vi "Read (Math).vi"(0 "VISA resource name":refnum<visa-resource-name>, 1 "Sample Count (1)":i32=1, 5 "Math Operation (0: Power)":u16(ring) items=["Power", "Offset Compensated Ohms", "Resistor Voltage Coefficient", "Varistor Alpha", "Custom Math Operation"], 7 "Custom Math Operation Name (\"Custom\")":string="Custom", 9 "Timeout (10000 ms)":i32=10000 format="%#.6g", 11 "error in (no error)":errorcluster, 12 "Output Mode (0: Fixed)":u16(ring) items=["Fixed", "Sweep", "List"]) -> (4 "VISA resource name out":refnum<visa-resource-name>, 6 "Math Results":dbl[](array[numeric]), 15 "error out":errorcluster)   [LabVIEW 2024, in "Keithley 24XX.lvlib"]
doc: "Initiates an acquisition and reads the result of the specified math operation."
uses:
  Keithley 24XX.lvlib
  Low Level/Fetch (Math).vi
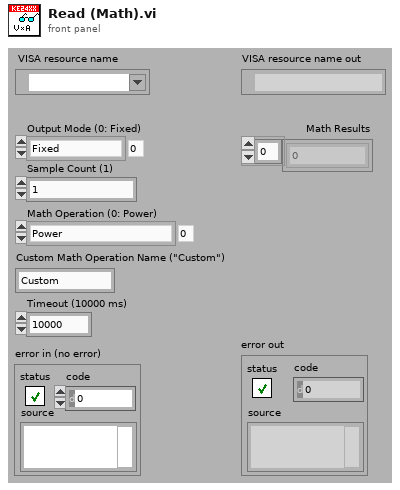
[diagram p1: front panel]
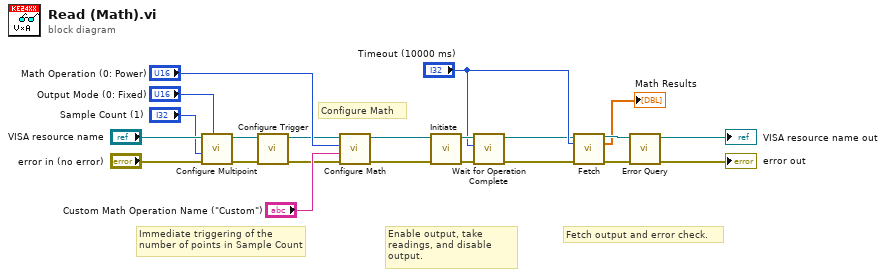
[diagram p0: block diagram]
diagram:
  # "Fetch output and error check."
  # "Enable output, take readings, and disable output."
  # "Configure Math"
  # "Immediate triggering of the number of points in Sample Count"
  n1 = call "Configure Multipoint.vi"("Output Mode (0: Fixed)"="Output Mode (0: Fixed)", "error in (no error)"="error in (no error)", "Trigger Count (1)"="Sample Count (1)", "VISA resource name"="VISA resource name") -> ("error out"=w7:errorcluster, "VISA resource name out"=w8:refnum<visa-resource-name>)  [unwired: 6 in]
  n2 = call "Configure Trigger.vi"("error in (no error)"=w7, "VISA resource name"=w8) -> ("error out"=w6:errorcluster, "VISA resource name out"=w5:refnum<visa-resource-name>)  [unwired: 8 in]
  n3 = call "Configure Math.vi"("error in (no error)"=w6, "Custom Math Operation Name (\"Custom\")"="Custom Math Operation Name (\"Custom\")", "Math Operation (0: Power)"="Math Operation (0: Power)", "VISA resource name"=w5) -> ("error out"=w3:errorcluster, "VISA resource name out"=w4:refnum<visa-resource-name>)  [unwired: 6 in]
  n4 = call "Initiate.vi"("error in (no error)"=w3, "VISA resource name"=w4) -> ("error out"=w14:errorcluster, "VISA resource name out"=w15:refnum<visa-resource-name>)  [unwired: 8 in]
  n5 = call "Wait for Operation Complete.vi"("error in (no error)"=w14, "Timeout (10000 ms)"="Timeout (10000 ms)", "VISA resource name"=w15) -> ("error out"=w1:errorcluster, "VISA resource name out"=w2:refnum<visa-resource-name>)  [unwired: 7 in]
  n6 = call-poly "Fetch.vi"("VISA resource name"=w2, "Timeout (10000 ms)"="Timeout (10000 ms)", "error in (no error)"=w1) -> ("VISA resource name out"=w19:refnum<visa-resource-name>, "Math Results"=→"Math Results":sgl[], "error out"=w20:errorcluster)  [unwired: 10 in]
  n7 = call "Error Query.vi"("error in (no error)"=w20, "VISA resource name"=w19) -> ("error out"=→"error out":errorcluster, "VISA resource name out"=→"VISA resource name out":refnum<visa-resource-name>)  [unwired: 6 in, 2 out]
